vi "Test TS Environment Manager - Profile Management.vi"() -> (0 "error out":errorcluster)   [LabVIEW 2025]
doc: "This VI tests profile management actions of the TS Environment manager (Add profile, read profile, delete profile) using a dummy INI file."
uses:
  src/Type Definitions/Profile--cluster.ctl
  src/Type Definitions/Architecture--enum.ctl
  <userlib>/_OpenG.lib/file/file.llb/File Exists - Scalar__ogtk.vi
  <vilib>/Utility/config.llb/Read Key (String).vi
  <vilib>/Utility/config.llb/Read Key (Path).vi
  <vilib>/addons/_JKI Toolkits/Caraya/classes/Assert/Assert.lvclass
  <userlib>/_OpenG.lib/file/file.llb/openg_file.lvlib
  <vilib>/Utility/config.llb/NI_LVConfig.lvlib
  src/Libraries/TS Environment Manager/TS Environment Manager.lvlib
  <vilib>/addons/_JKI Toolkits/Caraya/classes/Test/Test.lvclass
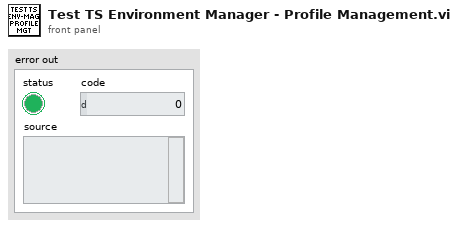
[diagram p1: front panel]
types:
  T1 = typedef "Architecture--enum.ctl" = enum16{"32bit", "64bit"}
  T2 = typedef "Profile--cluster.ctl" = cluster{"Name":string, "Version":string, "Architecture":T1, "Environment":path}
  T3 = typedef "NI_LVConfig.lvlib/Config Data RefNum.ctl" = refnum<k1>
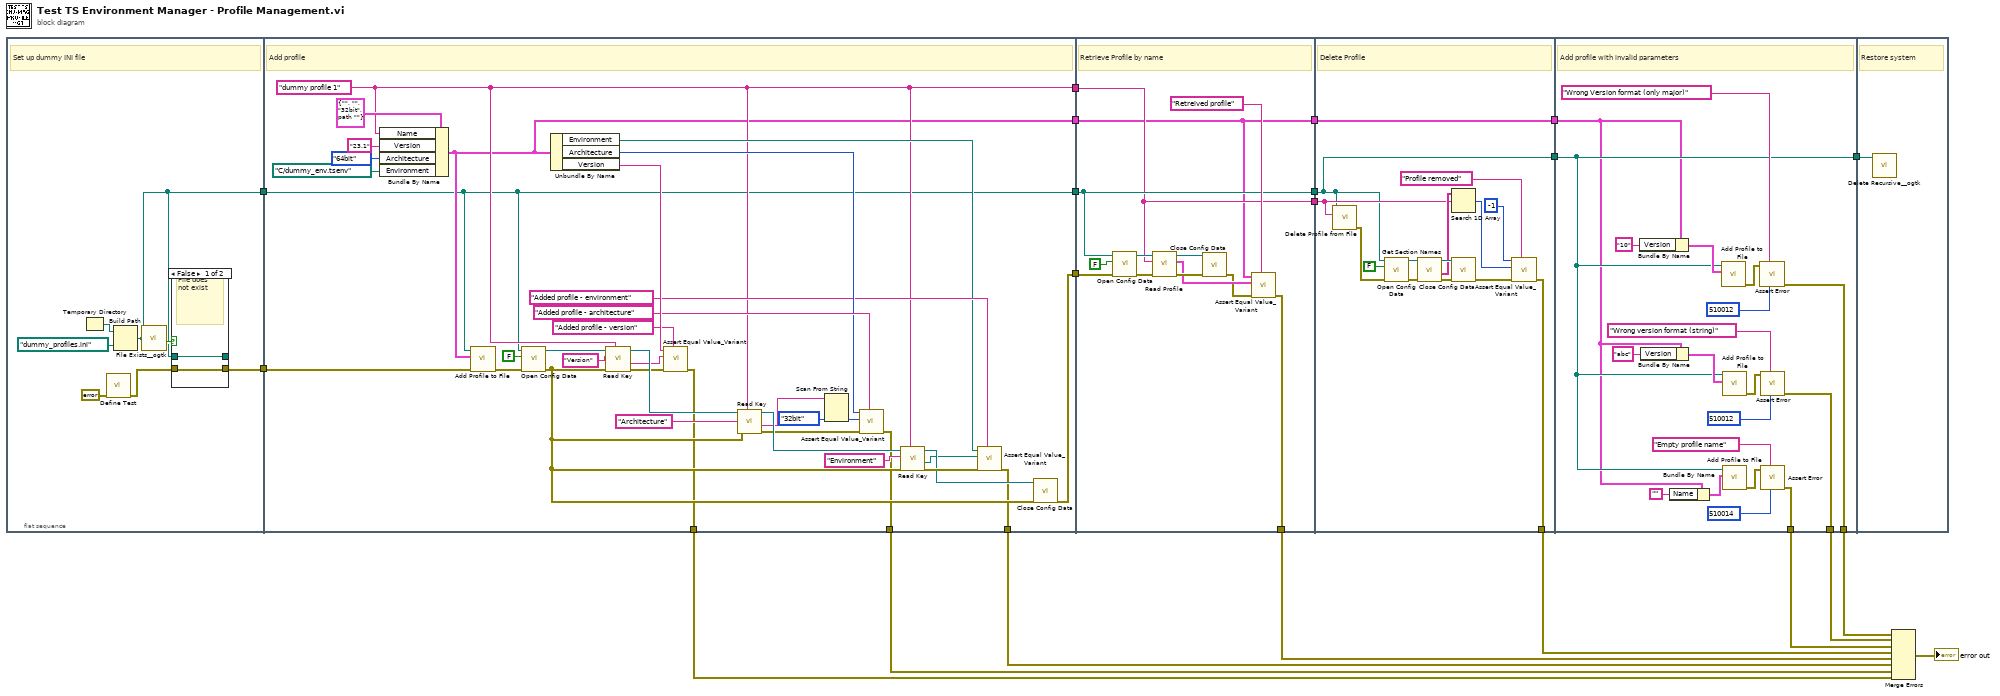
[diagram p0: block diagram]
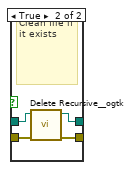
[diagram p2: hidden frame]
diagram:
  n1 = flat-sequence {
    tunnel: [w24] -> w21
    tunnel: [w25] -> w20
    tunnel: w21 -> [w44]
    tunnel: w20 -> [w41]
    tunnel: [w47] -> w19
    tunnel: [w42] -> w18
    tunnel: [w41] -> w17
    tunnel: [w39] -> w14
    tunnel: [w38] -> w11
    tunnel: [w37] -> w10
    tunnel: [w36] -> w9
    tunnel: w19 -> [w77]
    tunnel: w18 -> [w71]
    tunnel: w17 -> [w81]
    tunnel: [w77] -> w16
    tunnel: [w81] -> w15
    tunnel: w14 -> [w82]
    tunnel: [w72] -> w12
    tunnel: [w71] -> w4
    tunnel: w16 -> [w88]
    tunnel: w15 -> [w87]
    tunnel: [w87] -> w7
    tunnel: [w85] -> w13
    tunnel: [w84] -> w5
    tunnel: w4 -> [w84]
    tunnel: w7 -> [w101]
    tunnel: [w101] -> w6
    tunnel: w5 -> [w100]
    tunnel: [w110] -> w2
    tunnel: [w109] -> w3
    tunnel: [w102] -> w1
    tunnel: w6 -> [w119]
    frame #0 {
      # "Set up dummy INI file"
      n2 = Temporary Directory() -> (w28:path)
      n3 = call <vilib>:"Define Test.vi"("error in (no error)"=errorcluster {"status"=FALSE, "code"=0, "source"=""}) -> ("error out"=w22:errorcluster)  [unwired: 9 in, 1 out]
      n4 = Build Path(base path=w28, name or relative path=path "dummy_profiles.ini") -> (appended path=w25:path)
      n5 = call-poly <userlib>:"File Exists__ogtk.vi"("file path"=w25) -> ("exists"=w26:bool)  [unwired: 6 in, 1 out]
      n6 = case shown="False" w26 {
        tunnel: w25 -> [w30 w34]
        tunnel: [w29 w33] -> w24
        tunnel: [w30 w32] -> _
        tunnel: w22 -> [w29 w31]
        frame False {
          # "File does not exist"
        }
        frame True {
          # "Clean file if it exists"
          n7 = call <userlib>:"Delete Recursive__ogtk.vi"("error in (no error)"=w31, "Path"=w34) -> ("error out"=w33:errorcluster, "dup Path"=w32:path)  [unwired: 8 in]
        }
      }
    }
    frame #1 {
      w47 = "dummy profile 1" ("Name")
      # "Add profile"
      n8 = Bundle By Name(cluster=T2 {"Name"="", "Version"="", "Architecture"=enum."32bit", "Environment"=path ""} ("Profile"), "Name"=w47, "Version"="23.1", "Architecture"=Architecture--enum."64bit", "Environment"=path "C:/dummy_env.tsenv") -> (w42:T2)
      n9 = call "Add Profile to File.vi"("error in"=w44, "Profile"=w42, "File Path"=w41) -> ("error out"=w43:errorcluster)  [unwired: 8 in]
      n10 = call <vilib>:"Open Config Data.vi"("error in (no error)"=w43, "create file if necessary (T)"=FALSE, "configuration file path"=w41) -> ("error out"=w40:errorcluster, "refnum"=w65:T3)  [unwired: 6 in, 1 out]
      n11 = Unbundle By Name(w42) -> ("Environment"=w49:path, "Architecture"=w55:T1, "Version"=w61:string)
      n12 = call-poly <vilib>:"Read Key.vi"("section"=w47, "error in (no error)"=w40, "key"="Version", "refnum"=w65) -> ("error out"=w59:errorcluster, "value"=w60:string, "refnum out"=w63:T3)  [unwired: 4 in, 1 out]
      n13 = call <vilib>:"Assert Equal Value_Variant.vi"("Label"="Added profile - version", "error in (no error)"=w59, "Actual"=w60, "Expected"=w61) -> ("error out"=w36:errorcluster)  [unwired: 6 in, 1 out]
      n14 = call-poly <vilib>:"Read Key.vi"("section"=w47, "error in (no error)"=w40, "key"="Architecture", "refnum"=w63) -> ("error out"=w57:errorcluster, "value"=w54:string, "refnum out"=w62:T3)  [unwired: 4 in, 1 out]
      n15 = Scan From String(input string=w54, default 1=Architecture--enum."32bit" ("Architecture")) -> (output 1=w52:T1)  [unwired: 3 in, 3 out]
      n16 = call <vilib>:"Assert Equal Value_Variant.vi"("Label"="Added profile - architecture", "error in (no error)"=w57, "Actual"=w52, "Expected"=w55) -> ("error out"=w37:errorcluster)  [unwired: 6 in, 1 out]
      n17 = call-poly <vilib>:"Read Key.vi"("section"=w47, "error in (no error)"=w40, "key"="Environment", "refnum"=w62) -> ("error out"=w51:errorcluster, "value"=w35:path, "refnum out"=w48:T3)  [unwired: 4 in, 1 out]
      n18 = call <vilib>:"Assert Equal Value_Variant.vi"("Label"="Added profile - environment", "error in (no error)"=w51, "Actual"=w35, "Expected"=w49) -> ("error out"=w38:errorcluster)  [unwired: 6 in, 1 out]
      n19 = call <vilib>:"Close Config Data.vi"("error in (no error)"=w40, "refnum"=w48) -> ("error out"=w39:errorcluster)  [unwired: 8 in, 1 out]
    }
    frame #2 {
      # "Retrieve Profile by name"
      n20 = call <vilib>:"Open Config Data.vi"("error in (no error)"=w82, "create file if necessary (T)"=FALSE, "configuration file path"=w81) -> ("error out"=w79:errorcluster, "refnum"=w80:T3)  [unwired: 6 in, 1 out]
      n21 = call "Read Profile.vi"("error in"=w79, "Name"=w77, "File in"=w80) -> ("error out"=w75:errorcluster, "Profile"=w74:T2, "File out"=w76:T3)  [unwired: 6 in]
      n22 = call <vilib>:"Close Config Data.vi"("error in (no error)"=w75, "refnum"=w76) -> ("error out"=w73:errorcluster)  [unwired: 8 in, 1 out]
      n23 = call <vilib>:"Assert Equal Value_Variant.vi"("Label"="Retreived profile", "error in (no error)"=w73, "Actual"=w74, "Expected"=w71) -> ("error out"=w72:errorcluster)  [unwired: 6 in, 1 out]
    }
    frame #3 {
      # "Delete Profile"
      n24 = call "Delete Profile from File.vi"("Name"=w88, "Profile File"=w87) -> ("error out"=w86:errorcluster)  [unwired: 9 in]
      n25 = call <vilib>:"Open Config Data.vi"("error in (no error)"=w86, "create file if necessary (T)"=FALSE, "configuration file path"=w87) -> ("error out"=w97:errorcluster, "refnum"=w96:T3)  [unwired: 6 in, 1 out]
      n26 = call <vilib>:"Get Section Names.vi"("error in (no error)"=w97, "refnum"=w96) -> ("error out"=w95:errorcluster, "section names"=w93:string[], "refnum out"=w94:T3)  [unwired: 7 in]
      n27 = Search 1D Array(1D array=w93, element=w88) -> (index of element=w91:i32)  [unwired: 1 in]
      n28 = call <vilib>:"Close Config Data.vi"("error in (no error)"=w95, "refnum"=w94) -> ("error out"=w92:errorcluster)  [unwired: 8 in, 1 out]
      n29 = call <vilib>:"Assert Equal Value_Variant.vi"("Label"="Profile removed", "error in (no error)"=w92, "Actual"=w91, "Expected"=-1) -> ("error out"=w85:errorcluster)  [unwired: 6 in, 1 out]
    }
    frame #4 {
      # "Add profile with invalid parameters"
      n30 = Bundle By Name(cluster=w100, "Version"="10") -> (w117:T2)
      n31 = Bundle By Name(cluster=w100, "Version"="abc") -> (w113:T2)
      n32 = Bundle By Name(cluster=w100, "Name"="") -> (w106:T2)
      n33 = call "Add Profile to File.vi"("Profile"=w117, "File Path"=w101) -> ("error out"=w108:errorcluster)  [unwired: 9 in]
      n34 = call "Add Profile to File.vi"("Profile"=w113, "File Path"=w101) -> ("error out"=w107:errorcluster)  [unwired: 9 in]
      n35 = call "Add Profile to File.vi"("Profile"=w106, "File Path"=w101) -> ("error out"=w103:errorcluster)  [unwired: 9 in]
      n36 = call <vilib>:"Assert Error.vi"("error code (1)"=510012, "Label"="Wrong Version format (only major)", "Error?"=w108) -> ("error out"=w109:errorcluster)  [unwired: 7 in, 1 out]
      n37 = call <vilib>:"Assert Error.vi"("error code (1)"=510012, "Label"="Wrong version format (string)", "Error?"=w107) -> ("error out"=w110:errorcluster)  [unwired: 7 in, 1 out]
      n38 = call <vilib>:"Assert Error.vi"("error code (1)"=510014, "Label"="Empty profile name", "Error?"=w103) -> ("error out"=w102:errorcluster)  [unwired: 7 in, 1 out]
    }
    frame #5 {
      # "Restore system"
      n39 = call <userlib>:"Delete Recursive__ogtk.vi"("Path"=w119) -> ()  [unwired: 9 in, 2 out]
    }
  }
  n40 = Merge Errors(w3, w2, w1, w13, w12, w11, w10, w9) -> (→"error out":errorcluster)
